vi "writeVideoConfig.vi"() -> ()   [LabVIEW 2020]
uses:
  AimingBeamVideoConfig.ctl
  <vilib>/Utility/config.llb/Write Key (I32).vi
  <vilib>/Utility/config.llb/Write Key (Boolean).vi
  <vilib>/Utility/config.llb/Write Key (Double).vi
  <vilib>/Utility/config.llb/NI_LVConfig.lvlib
panel:
  out "file path":path
  out "error out":errorcluster
  in  "error in (no error)":errorcluster
  in  "Aiming Beam Config":T1={"DeCon Channel"=enum."1", "Scale Bar"=FALSE, "Scale Low"=3.0, "Scale High"=8.0, "ANSI"=20.0, "Radius"=1.0, "3D?"=FALSE, "Firefly?"=FALSE, "Pentero?"=FALSE}
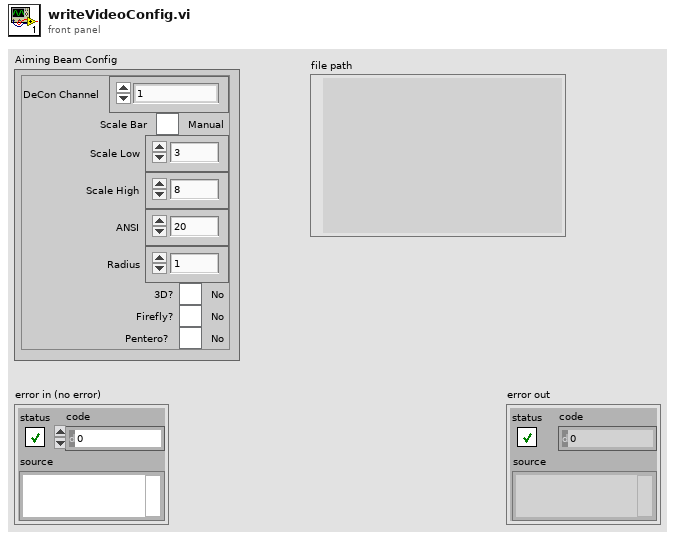
[diagram p1: front panel]
types:
  T1 = typedef "AimingBeamVideoConfig.ctl" = cluster{"DeCon Channel":enum16{"1", "2", "3"}, "Scale Bar":bool, "Scale Low":dbl, "Scale High":dbl, "ANSI":dbl, "Radius":dbl, "3D?":bool, "Firefly?":bool, "Pentero?":bool}
  T2 = typedef "NI_LVConfig.lvlib/Config Data RefNum.ctl" = refnum<k1>
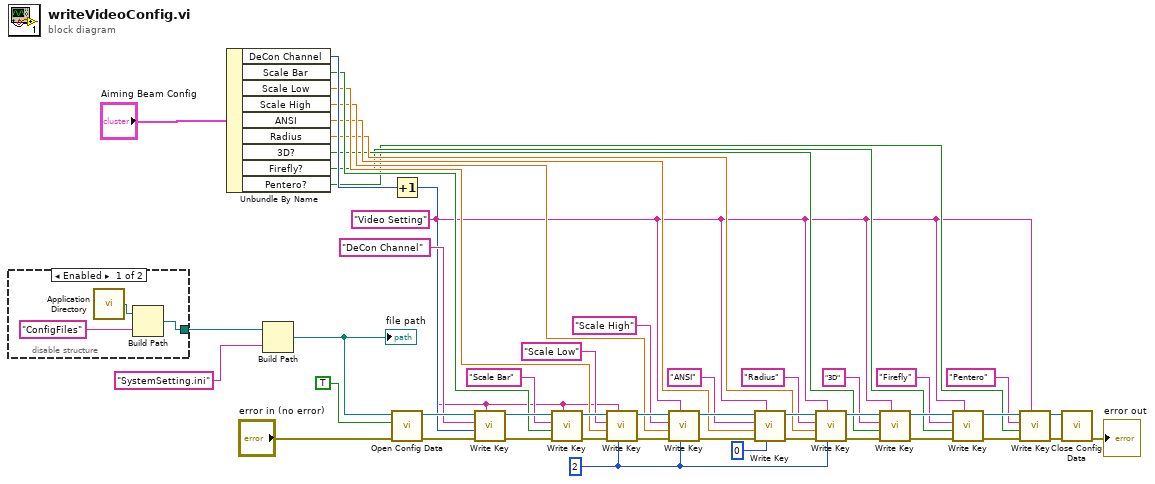
[diagram p0: block diagram]
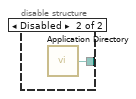
[diagram p2: hidden frame]
diagram:
  w1 = i16 2 ("precision (6)")
  w3 = "Video Setting" ("section")
  n1 = disable-structure shown="Enabled" {
    disable-tunnel: [w50 w53] -> w47
    frame Enabled {
      n2 = call <vilib>:"Application Directory.vi"() -> ("Application Directory"=w52:path)
      n3 = Build Path(base path=w52, name or relative path="ConfigFiles") -> (appended path=w50:path)
    }
    frame Disabled {
      n4 = call <vilib>:"Application Directory.vi"() -> ("Application Directory"=w53:path)
    }
  }
  n5 = Unbundle By Name("Aiming Beam Config") -> ("DeCon Channel"=w41:enum16{"1", "2", "3"}, "Scale Bar"=w35:bool, "Scale Low"=w31:dbl, "Scale High"=w28:dbl, "ANSI"=w23:dbl, "Radius"=w19:dbl, "3D?"=w15:bool, "Firefly?"=w11:bool, "Pentero?"=w7:bool)
  n6 = Build Path(base path=w47, name or relative path="SystemSetting.ini") -> (appended path=w45:path)
  "file path" <- w45
  n7 = Increment(x=w41) -> (x+1=w40:enum16{"1", "2", "3"})
  n8 = call <vilib>:"Open Config Data.vi"("error in (no error)"="error in (no error)", "create file if necessary (T)"=TRUE, "configuration file path"=w45) -> ("error out"=w39:errorcluster, "refnum"=w44:T2)  [unwired: 6 in, 1 out]
  n9 = call-poly <vilib>:"Write Key.vi"("section"=w3, "error in (no error)"=w39, "value"=w40, "key"="DeCon Channel", "refnum"=w44) -> ("error out"=w37:errorcluster, "refnum out"=w38:T2)  [unwired: 4 in, 1 out]
  n10 = call-poly <vilib>:"Write Key.vi"("section"=w3, "error in (no error)"=w37, "value"=w35, "key"="Scale Bar", "refnum"=w38) -> ("error out"=w33:errorcluster, "refnum out"=w34:T2)  [unwired: 4 in, 1 out]
  n11 = call-poly <vilib>:"Write Key.vi"("precision (6)"=w1, "section"=w3, "error in (no error)"=w33, "value"=w31, "key"="Scale Low", "refnum"=w34) -> ("error out"=w27:errorcluster, "refnum out"=w30:T2)  [unwired: 3 in, 1 out]
  n12 = call-poly <vilib>:"Write Key.vi"("precision (6)"=w1, "section"=w3, "error in (no error)"=w27, "value"=w28, "key"="Scale High", "refnum"=w30) -> ("error out"=w25:errorcluster, "refnum out"=w26:T2)  [unwired: 3 in, 1 out]
  n13 = call-poly <vilib>:"Write Key.vi"("precision (6)"=i16 0, "section"=w3, "error in (no error)"=w25, "value"=w23, "key"="ANSI", "refnum"=w26) -> ("error out"=w21:errorcluster, "refnum out"=w22:T2)  [unwired: 3 in, 1 out]
  n14 = call-poly <vilib>:"Write Key.vi"("precision (6)"=w1, "section"=w3, "error in (no error)"=w21, "value"=w19, "key"="Radius", "refnum"=w22) -> ("error out"=w17:errorcluster, "refnum out"=w18:T2)  [unwired: 3 in, 1 out]
  n15 = call-poly <vilib>:"Write Key.vi"("section"=w3, "error in (no error)"=w17, "value"=w15, "key"="3D", "refnum"=w18) -> ("error out"=w13:errorcluster, "refnum out"=w14:T2)  [unwired: 4 in, 1 out]
  n16 = call-poly <vilib>:"Write Key.vi"("section"=w3, "error in (no error)"=w13, "value"=w11, "key"="Firefly", "refnum"=w14) -> ("error out"=w9:errorcluster, "refnum out"=w10:T2)  [unwired: 4 in, 1 out]
  n17 = call-poly <vilib>:"Write Key.vi"("section"=w3, "error in (no error)"=w9, "value"=w7, "key"="Pentero", "refnum"=w10) -> ("error out"=w5:errorcluster, "refnum out"=w6:T2)  [unwired: 4 in, 1 out]
  n18 = call <vilib>:"Close Config Data.vi"("error in (no error)"=w5, "refnum"=w6) -> ("error out"=→"error out":errorcluster)  [unwired: 8 in, 1 out]
